vi "Open Data Log File.vi"(8 "error in":errorcluster, 9 "File Properties":T3[](array[typedef]), 10 "Channel Groups":T1[](array[typedef]), 11 "Data Log File Path":path) -> (0 "error out":errorcluster, 2 "File Start Time":timestamp, 3 "tdms file out":refnum<k34>)   [LabVIEW 2027, in "Embedded Data Logger Engine.lvlib"]
uses:
  Embedded Data Logger Engine.lvlib
  Property Specification.ctl
  Group Logging Specification.ctl
  Group Buffer Data.ctl
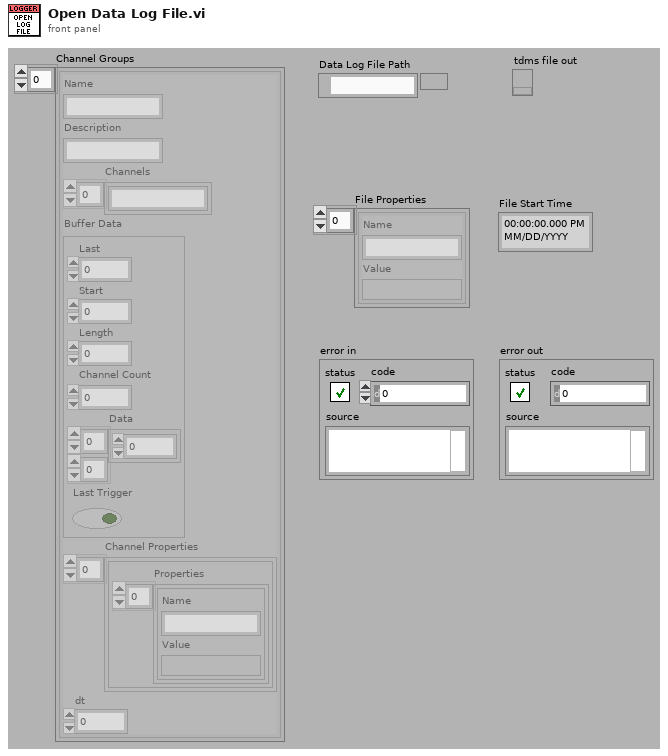
[diagram p1: front panel]
types:
  T1 = typedef "Embedded Data Logger Engine.lvlib/Group Logging Specification.ctl" = cluster{"Name":string, "Description":string, "Channels":string[], "Buffer Data":T2, "Channel Properties":cluster{"Properties":T3[]}[], "dt":dbl}
  T2 = typedef "Embedded Data Logger Engine.lvlib/Group Buffer Data.ctl" = cluster{"Last":i32, "Start":i32, "Length":i32, "Channel Count":i32, "Data":dbl[][], "Last Trigger":bool}
  T3 = typedef "Embedded Data Logger Engine.lvlib/Property Specification.ctl" = cluster{"Name":string, "Value":variant}
  T4 = enum16{"open", "open or create", "create or replace", "create", "open (read-only)"}
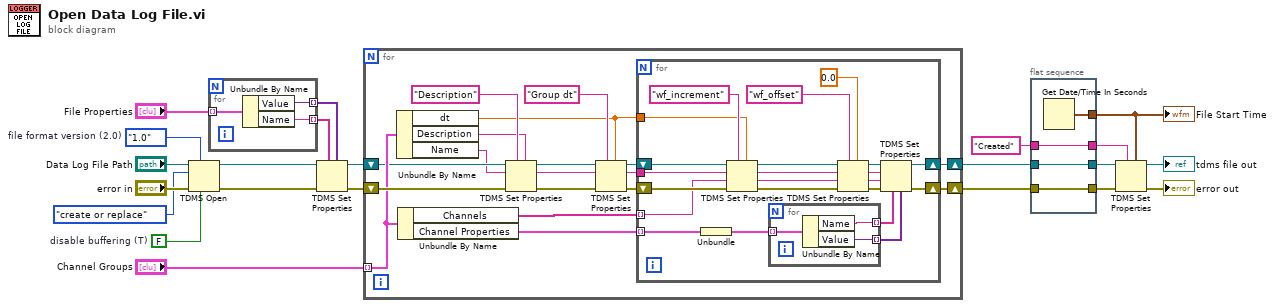
[diagram p0: block diagram]
diagram:
  w19 = FALSE  # disable buffering (T)
  w18 = enum16{"1.0", "2.0"}."1.0"  # file format version (2.0)
  n1 = TDMS Open(6:w19, 7:w18, 8:"error in", 10:T4."create or replace" ("operation (0:open)"), 11:"Data Log File Path") -> (0:w16:errorcluster, 3:w15:refnum<k34>)  [unwired: 2 in]
  n2 = for {
    tunnel: "File Properties" -> [w25] mode=indexing
    tunnel: [w24] -> w11 mode=indexing
    tunnel: [w23] -> w10 mode=indexing
    n3 = Unbundle By Name(w25) -> ("Value"=w23:variant, "Name"=w24:string)
  }
  n4 = TDMS Set Properties(5:w10, 7:w11, 8:w16, 11:w15) -> (0:w12:errorcluster, 3:w13:refnum<k34>)  [unwired: 1 in, 3 out]
  n5 = for {
    shift-right: [w42] -> w9
    shift-left: w12 -> [w43]
    shift-right: [w41] -> w5
    shift-left: w13 -> [w38]
    tunnel: "Channel Groups" -> [w39] mode=indexing
    n6 = Unbundle By Name(w39) -> ("dt"=w26:dbl, "Description"=w35:string, "Name"=w37:string)
    n7 = Unbundle By Name(w39) -> ("Channels"=w40:string[], "Channel Properties"=w34:cluster{"Properties":T3[]}[])
    n8 = TDMS Set Properties(5:w35, 7:"Description", 8:w43, 10:w37, 11:w38) -> (0:w28:errorcluster, 2:w32:string, 3:w33:refnum<k34>)  [unwired: 1 in, 1 out]
    n9 = TDMS Set Properties(5:w26, 7:"Group dt", 8:w28, 10:w32, 11:w33) -> (0:w29:errorcluster, 2:w30:string, 3:w31:refnum<k34>)  [unwired: 1 in, 1 out]
    n10 = for {
      shift-right: [w61] -> w42
      shift-left: w29 -> [w64]
      shift-right: [w62] -> w41
      shift-left: w31 -> [w65]
      tunnel: w30 -> [w63]
      tunnel: w40 -> [w59] mode=indexing
      tunnel: w34 -> [w58] mode=indexing
      tunnel: w26 -> [w48]
      n11 = Unbundle(w58) -> ("Properties"=w46:T3[])
      n12 = TDMS Set Properties(5:w48, 7:"wf_increment", 8:w64, 9:w59, 10:w63, 11:w65) -> (0:w55:errorcluster, 1:w49:string, 2:w50:string, 3:w56:refnum<k34>)
      n13 = for {
        tunnel: w46 -> [w68] mode=indexing
        tunnel: [w67] -> w45 mode=indexing
        tunnel: [w66] -> w44 mode=indexing
        n14 = Unbundle By Name(w68) -> ("Name"=w67:string, "Value"=w66:variant)
      }
      n15 = TDMS Set Properties(5:0.0 ("dt"), 7:"wf_offset", 8:w55, 9:w49, 10:w50, 11:w56) -> (0:w53:errorcluster, 1:w51:string, 2:w52:string, 3:w54:refnum<k34>)
      n16 = TDMS Set Properties(5:w44, 7:w45, 8:w53, 9:w51, 10:w52, 11:w54) -> (0:w61:errorcluster, 3:w62:refnum<k34>)  [unwired: 2 out]
    }
  }
  n17 = flat-sequence {
    tunnel: [w72] -> w1
    tunnel: w9 -> [w70]
    tunnel: [w70] -> w6
    tunnel: w5 -> [w71]
    tunnel: [w71] -> w4
    tunnel: [w69] -> w3
    tunnel: "Created" ("Name") -> [w69]
    frame #0 {
      n18 = Get Date/Time In Seconds() -> (seconds since 1Jan1904=w72:timestamp)
    }
  }
  n19 = TDMS Set Properties(5:w1, 7:w3, 8:w6, 11:w4) -> (0:→"error out":errorcluster, 3:→"tdms file out":refnum<k34>)  [unwired: 1 in, 3 out]
  "File Start Time" <- w1
